vi "ValidateModeArray.vi"() -> (0 "Valid?":bool)   [LabVIEW 2012, in "FTC.lvlib" / "Remote Interface.lvlib"]
uses:
  Remote Interface.lvlib
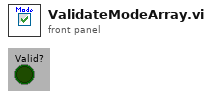
[diagram p1: front panel]
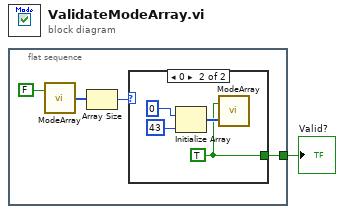
[diagram p0: block diagram]
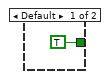
[diagram p2: hidden frame]
diagram:
  n1 = flat-sequence {
    tunnel: [w2] -> w1
    frame #0 {
      n2 = call "ModeArray.vi"("Write?"=FALSE) -> ("Array"=w4:u16[])  [unwired: 1 in]
      n3 = Array Size(array=w4) -> (size(s)=w3:i32)
      n4 = case shown="0" w3 {
        tunnel: [TRUE ("Write?") w8] -> w2
        frame Default {
        }
        frame 0 {
          w8 = TRUE ("Write?")
          n5 = Initialize Array(u16 0, 43) -> (w9:u16[])
          n6 = call "ModeArray.vi"("Write Array"=w9, "Write?"=w8) -> ()  [unwired: 1 out]
        }
      }
    }
  }
  "Valid?" <- w1
